vi "_Nitsuki_TPD_control_send.vi"(10 "send":string, 11 "control IP":string) -> (2 "Their Response:":string caption="応答：", 3 "control IP  2":string)   [LabVIEW 2017]
panel:
  out "error out":errorcluster caption="エラー出力"
  out "文字列":string
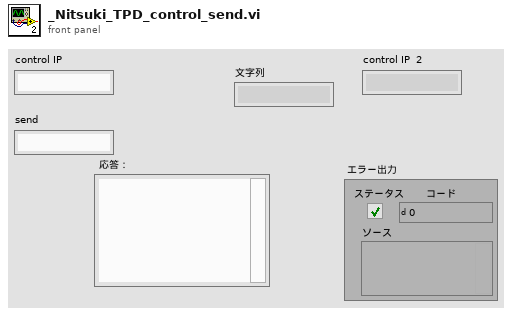
[diagram p1: front panel]
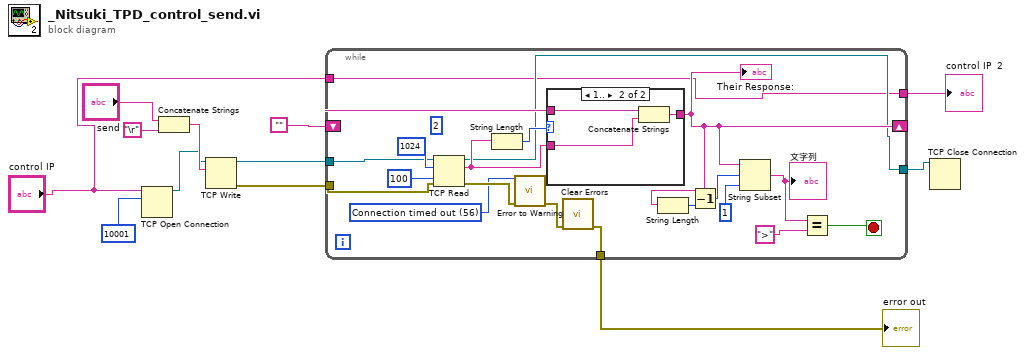
[diagram p0: block diagram]
diagram:
  n1 = TCP Open Connection(address="control IP", remote port or service name=10001) -> (connection ID=w4:refnum<k5>)  [unwired: 3 in, 1 out]
  n2 = Concatenate Strings("send", "\r") -> (w7:string)
  n3 = TCP Write(connection ID=w4, data in=w7) -> (connection ID out=w12:refnum<k5>, error out=w10:errorcluster)  [unwired: 2 in, 1 out]
  n4 = while {
    tunnel: w12 -> [w31]
    shift-right: [w23] -> _
    shift-left: "" -> [w27]
    tunnel: w10 -> [w25]
    tunnel: [w16] -> w6
    tunnel: [w14] -> w3
    tunnel: "control IP" -> [w13]
    tunnel: [w13] -> w1
    stop <- w18 stop-if-true
    (unwired) 2
    w29 = 56 items=["No Error", "Argument Error", "Memory Full", "Out of Zone", "End of File", "File Already Open", "Generic File IO Error", "File Not Found", "File Permission Error", "Disk Full", "Duplicate Path", "Too Many Files Open", "Not Enabled", "Resource File Not Found", "Cannot Add Resource", "Resource Not Found", "Image Not Found", "Image Memory Error", "Pen Does Not Exist", "Config Bad Type", "Config Token Not Found", "Config Parse Error", "Config Memory Error", "Bad External Code Format", "Bad External Code Offset", "External Code Not Present", "Null Window", "Destroy Window Mixup", "Null Menu", "Print Aborted", "Bad Print Record", "Print Driver Error", "Windows Error During Print", "Memory Error During Print", "Print Dialog Error", "Generic Print Error", "Invalid Device Refnum", "Device Not Found", "Device Parameter Error", "Device Unit Error", "Can't Open Device", "Device Call Aborted", "Generic Error", "Cancelled By User", "Object ID Too Low", "Object ID Too High", "Object Not In Heap", "Unknown Heap", "Bad DefProc ID", "DefProc Not In Table", "Message Out Of Range", "Null Method", "Unknown Message", "Manager Call Not Supported", "Bad address", "Connection In progress", "Connection timed out", "Connection is already in progress", "Network attribute not supported", "Network error", "Address in use", "System out of memory", "Connection aborted", "Connection refused", "Connection is not connected", "Connection is already connected", "Connection closed", "Initialize error (interapplication manager)", "Bad occurrence", "Wait on unbound occurrence handler", "Occurrence queue overflow", "Bad path", "Semaphore not signaled", "Unrecognized type (interapplication manager)"] ("1st Error to Convert")
    n5 = TCP Read(connection ID=w31, bytes to read=1024, error in (no error)=w25, 9:100) -> (connection ID out=w14:refnum<k5>, data out=w26:string, error out=w30:errorcluster)  [unwired: 1 in]
    n6 = String Length(string=w26) -> (length=w28:i32)
    n7 = call <vilib>:"Error to Warning.vi"("1st Error to Convert"=w29, "error in"=w30) -> ("warning out"=w17:errorcluster)  [unwired: 13 in]
    n8 = case shown="1.." w28 {
      tunnel: w26 -> [_ w34]
      tunnel: w27 -> [w33 w36]
      tunnel: [w33 w35] -> w23
      frame ..0 {
      }
      frame 1.. {
        n9 = Concatenate Strings(w36, w34) -> (w35:string)
      }
    }
    "Their Response:" <- w23
    n10 = call <vilib>:"Clear Errors.vi"("error in (no error)"=w17) -> ("error out"=w16:errorcluster)  [unwired: 5 in, 1 out]
    n11 = String Length(string=w23) -> (length=w24:i32)
    n12 = Decrement(x=w24) -> (x-1=w22:i32)
    n13 = String Subset(string=w23, offset (0)=w22, length (rest)=1) -> (substring=w20:string)
    "文字列" <- w20
    n14 = Equal?(x=w20, y=">") -> (x = y?=w18:bool)
  }
  "error out" <- w6
  "control IP  2" <- w1
  n15 = TCP Close Connection(connection ID=w3) -> ()  [unwired: 2 in, 2 out]
